vi "SetLightingConditions.vi"(4 "Bus Tape Gain":dbl, 6 "Si Gain":dbl, 10 "Spotlights Refnum":refnum<vi>, 11 "Coaxial Light Refnum":refnum<vi>) -> (1 "Assigned Camera Gain":dbl, 2 "Spotlights on?":bool, 3 "Coaxial on?":bool)   [LabVIEW 2016]
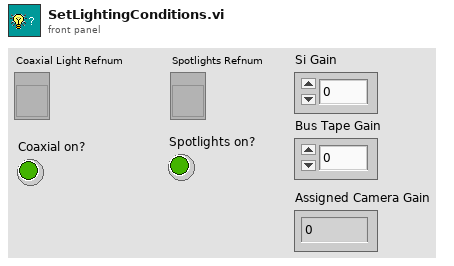
[diagram p1: front panel]
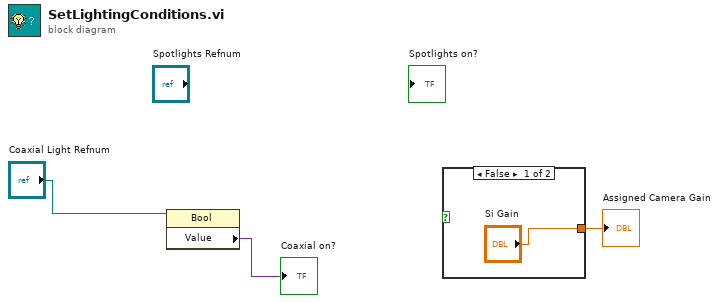
[diagram p0: block diagram]
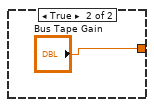
[diagram p2: hidden frame]
diagram:
  n1 = property class="Bool"(reference="Coaxial Light Refnum") -> ("Value"=→"Coaxial on?":variant)  [unwired: 1 in, 2 out]
  n2 = case shown="False" w3 {
    tunnel: ["Si Gain" "Bus Tape Gain"] -> w4
    frame False {
    }
    frame True {
    }
  }
  "Assigned Camera Gain" <- w4
